vi "niRFUtil MT UTIL Generate Integer Interpolation Filter.vi"(11 "interpolation factor":i32=1) -> (1 "filter coefficients out":T1 min=0 max=127 format="%.2f", 2 "total length":i32, 3 "polyphase filter out (2D)":sgl[][](array[numeric]), 5 "polyphase filter out (1D)":sgl[](array[numeric]))   [LabVIEW 2015, in "niRFUtil.lvlib"]
uses:
  niRFUtil.lvlib
  Includes/niRFUtil INC Real Array.ctl
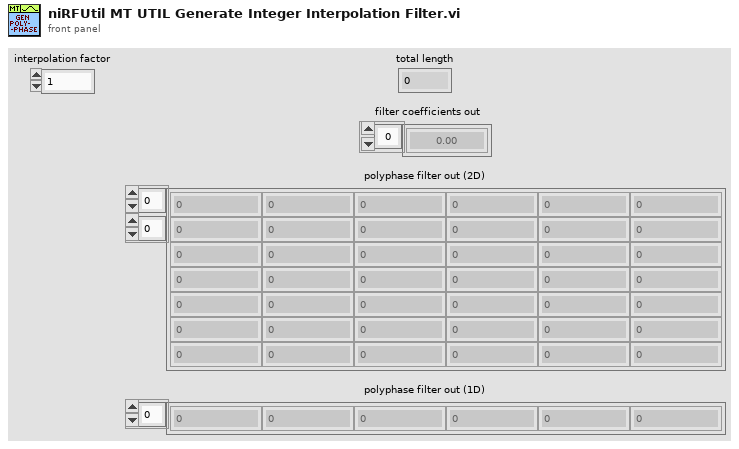
[diagram p1: front panel]
types:
  T1 = typedef "niRFUtil.lvlib/niRFUtil INC Real Array.ctl" = sgl[]
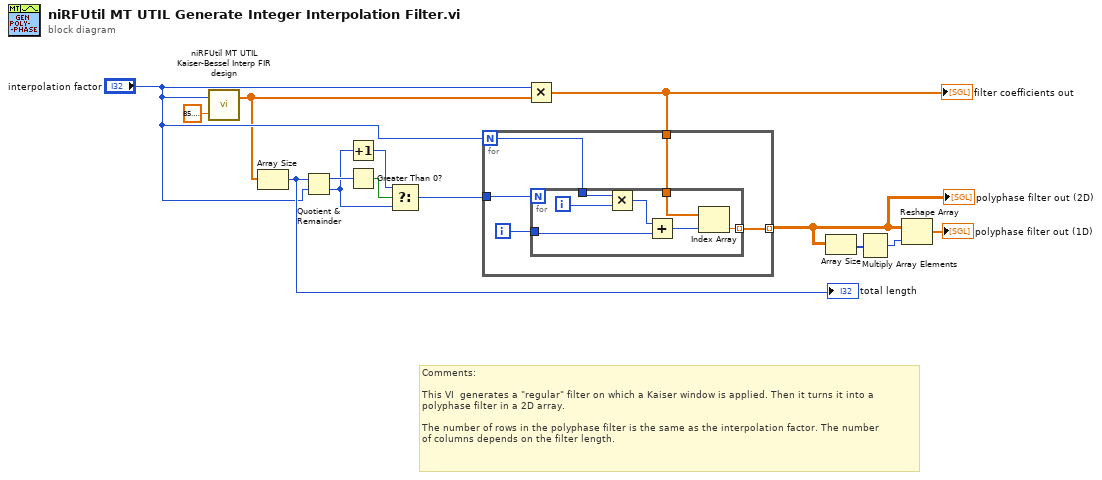
[diagram p0: block diagram]
diagram:
  # "Comments:\n\nThis VI  generates a \"regular\" filter on which a Kaiser window is applied. Then it turns it into a\npolyphase filter in a 2D array.\n\nThe number of rows in the polyphase filter is the same as the interpolation factor. The number\nof columns depends on the filter length."
  n1 = call "niRFUtil MT UTIL Kaiser-Bessel Interp FIR design.vi"("Stop Attenuation"=85.00000000000051, "interpolation factor"="interpolation factor") -> ("h"=w1:T1)  [unwired: 1 in]
  n2 = Array Size(array=w1) -> (size(s)=w5:i32)
  "total length" <- w5
  n3 = Quotient & Remainder(x=w5, y="interpolation factor") -> (x-y*floor(x/y)=w13:i32, floor(x/y)=w12:i32)
  n4 = Increment(x=w12) -> (x+1=w11:i32)
  n5 = Greater Than 0?(x=w13) -> (x > 0?=w14:bool)
  n6 = Select(t=w11, s=w14, f=w12) -> (s? t:f=w10:i32)
  n7 = Multiply(x="interpolation factor", y=w1) -> (x*y=w4:T1)
  "filter coefficients out" <- w4
  n8 = for {
    N: "interpolation factor" -> [w17]
    tunnel: w10 -> [w19]
    tunnel: w4 -> [w16]
    tunnel: [w15] -> w6 mode=indexing
    i -> [w18]
    n9 = for {
      N: w19 -> [_]
      tunnel: w18 -> [w23]
      tunnel: w17 -> [w25]
      tunnel: w16 -> [w21]
      tunnel: [w20] -> w15 mode=indexing
      i -> [w26]
      n10 = Multiply(x=w25, y=w26) -> (x*y=w24:i32)
      n11 = Add(x=w24, y=w23) -> (x+y=w22:i32)
      n12 = Index Array(array=w21, index=w22) -> (element=w20:sgl)
    }
  }
  "polyphase filter out (2D)" <- w6
  n13 = Array Size(array=w6) -> (size(s)=w8:i32[])
  n14 = Multiply Array Elements(1:w8) -> (0:w9:i32)
  n15 = Reshape Array(w6, w9) -> (→"polyphase filter out (1D)":sgl[])
